vi "HDF5 append data.vi"   [LabVIEW 2013]
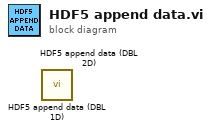
[diagram p0: block diagram]
diagram:
  n1 = call "HDF5 append data (DBL 1D).vi"() -> ()  [unwired: 10 in, 2 out]
  n2 = call "HDF5 append data (DBL 2D).vi"() -> ()  [unwired: 10 in, 2 out]
